vi "Close.vi"(8 "error in (no error)":errorcluster, 11 "Study Base in":refnum<class "Study Base.lvclass">) -> (0 "error out":errorcluster, 3 "Study Base out":refnum<class "Study Base.lvclass">)   [LabVIEW 2023, in "HAL GOOP4.lvlib" / "Study Base.lvclass"]
uses:
  Study Base.lvclass
  Study Base.lvclass/Study Base.ctl
  Measure and Stimulus Subsystems/Measure and Stimulus Subsystems.lvclass
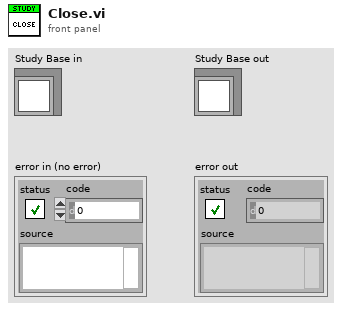
[diagram p1: front panel]
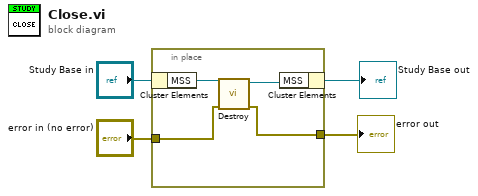
[diagram p0: block diagram]
diagram:
  n1 = in-place "In Place Element Structure" {
    in-place-border: "error in (no error)" -> [w6]
    in-place-border: [w5] -> w1
    n2 = in-place-cluster #1("Study Base in") -> ("MSS"=w8:refnum<class "Measure and Stimulus Subsystems.lvclass">)
    n3 = call "Destroy.vi"("Error In"=w6, "reference in"=w8) -> ("Error Out"=w5:errorcluster, "reference out"=w7:refnum<class "Measure and Stimulus Subsystems.lvclass">)  [unwired: 8 in]
    n4 = in-place-cluster #1("MSS"=w7) -> (→"Study Base out":refnum<class "Study Base.lvclass">)
  }
  "error out" <- w1
